vi "Write Setting.vi"(8 "error in":errorcluster, 10 "Setting":dbl, 11 "PRM in":refnum<class "PRM.lvclass">) -> (0 "error out":errorcluster, 3 "PRM out":refnum<class "PRM.lvclass">)   [LabVIEW 2019, in "PRM.lvlib" / "PRM.lvclass"]
uses:
  Library/PRM.lvclass
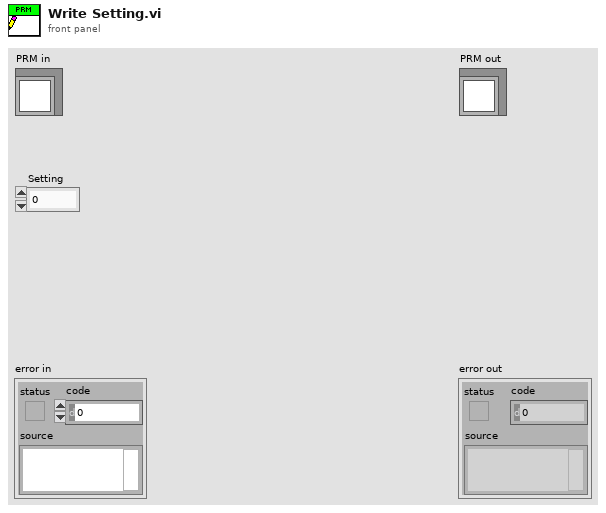
[diagram p1: front panel]
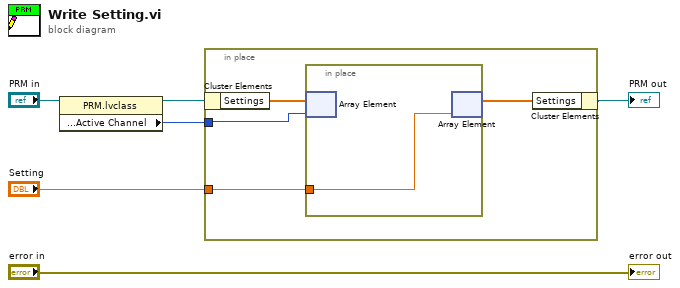
[diagram p0: block diagram]
diagram:
  n1 = property class="PRM.lvclass"(reference="PRM in") -> (reference out=w5:refnum<class "PRM.lvclass">, "Accessors:Settings:Active Channel"=w2:u32)  [unwired: 1 in, 1 out]
  n2 = in-place {
    in-place-border: "Setting" -> [w9]
    in-place-border: w2 -> [w7]
    n3 = in-place-cluster #1(w5) -> ("Settings"=w10:dbl[])
    n4 = in-place {
      in-place-border: w9 -> [w11]
      n5 = in-place-array #2(w10, w7) -> ()  [unwired: 1 out]
      n6 = in-place-array #2(w11) -> (w8:dbl[])  [unwired: 1 out]
    }
    n7 = in-place-cluster #1("Settings"=w8) -> (→"PRM out":refnum<class "PRM.lvclass">)
  }
  "error out" <- "error in"
